vi "DemoSubClass1_Create.vi"(0 "reference in":refnum<class "DemoSubClass1.lvclass">, 5 "error in (no error)":errorcluster) -> (14 "reference out":refnum<class "DemoSubClass1.lvclass">, 19 "error out":errorcluster)   [LabVIEW 2016, in "DemoSubClass1.lvclass"]
uses:
  <vilib>/addons/GOOPUtility/_Demo/GOOPUtil_Demo/DemoSubClass1_class/DemoSubClass1.lvclass
  C:/Program Files (x86)/National Instruments/LabVIEW 2016/vi.lib/addons/GOOPUtility/_Demo/GOOPUtil_Demo/DemoClass1_class/DemoClass1.lvclass
  <vilib>/addons/GOOPUtility/_Demo/GOOPUtil_Demo/DemoClass1_class/DemoClass1.lvclass
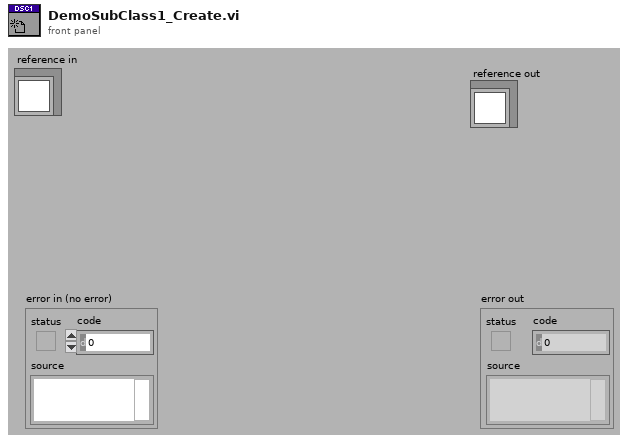
[diagram p1: front panel]
types:
  T1 = enum16{"Create", "Create or look up existing", "Look up existing"}
  T2 = typedef "DemoSubClass1.lvclass/ObjectAttributes.ctl" = cluster{"Base class":T3}
  T3 = typedef "DemoClass1.lvclass/ObjectAttributes.ctl" = cluster{"Attribute1":dbl}
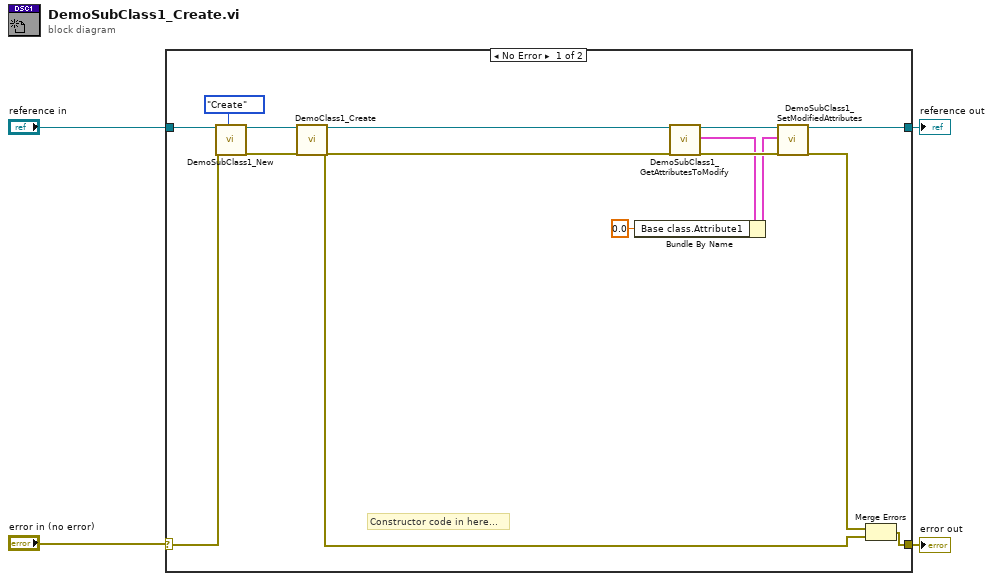
[diagram p0: block diagram]
diagram:
  n1 = case shown="No Error" "error in (no error)" {
    selector: "error in (no error)" -> [w17 w21]
    tunnel: [w10 w21] -> w3
    tunnel: [w15 w20] -> w2
    tunnel: "reference in" -> [w7 w20]
    frame No Error {
      # "Constructor code in here..."
      n2 = call <vilib>:"DemoSubClass1_New.vi"("reference in"=w7, "error in (no error)"=w17, "Create method"=T1."Create") -> ("reference out"=w12:refnum<class "DemoSubClass1.lvclass">, "error out"=w16:errorcluster)  [unwired: 13 in, 2 out]
      n3 = call <vilib>:"DemoClass1_Create.vi"("reference in"=w12, "error in (no error)"=w16) -> ("reference out"=w11:refnum<class "DemoSubClass1.lvclass">, "error out"=w8:errorcluster)  [unwired: 16 in]
      n4 = call <vilib>:"DemoSubClass1_GetAttributesToModify.vi"("reference in"=w11, "error in (no error)"=w8) -> ("reference out"=w19:refnum<class "DemoSubClass1.lvclass">, "Attributes"=w14:T2, "error out"=w18:errorcluster)  [unwired: 14 in, 1 out]
      n5 = Bundle By Name(cluster=w14, "Base class.Attribute1"=0.0) -> (w13:T2)
      n6 = call <vilib>:"DemoSubClass1_SetModifiedAttributes.vi"("reference in"=w19, "Attributes"=w13, "error in (no error)"=w18) -> ("reference out"=w15:refnum<class "DemoSubClass1.lvclass">, "error out"=w9:errorcluster)  [unwired: 15 in]
      n7 = Merge Errors(w9, w8) -> (w10:errorcluster)
    }
    frame Error {
    }
  }
  "error out" <- w3
  "reference out" <- w2
